vi "get property indeces.vi"(8 "error in":errorcluster, 10 "channels":refnum<class "TBM channel.lvclass">[](array[class]), 11 "data dictionary in":refnum<class "data dictionary.lvclass">) -> (0 "error out":errorcluster, 2 "File Property Indeces":i32[](array[numeric]), 3 "data dictionary out":refnum<class "data dictionary.lvclass">)   [LabVIEW 2015, in "TDMS datalogger runtime.lvclass"]
uses:
  TDMS datalogger runtime.lvclass
  <vilib>/NI/Tag Bus Module Framework/channel/TBM channel.lvclass
  <vilib>/NI/Tag Bus/dictionary/data dictionary.lvclass
  <vilib>/NI/Tag Bus/tag/tag descriptor.lvclass/tag descriptor.ctl
  <vilib>/NI/Tag Bus/tag/read tag name.vi
  <vilib>/NI/Tag Bus/tag/read data type.vi
  <vilib>/NI/Tag Bus/dictionary/locate tag.vi
  <vilib>/NI/Tag Bus/tag/tag descriptor.lvclass
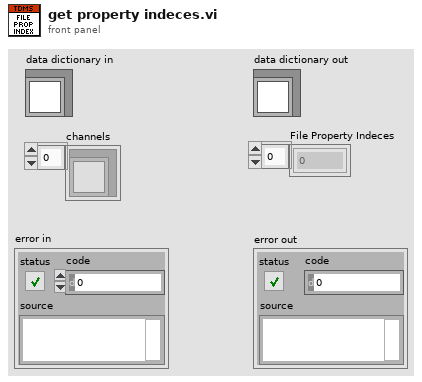
[diagram p1: front panel]
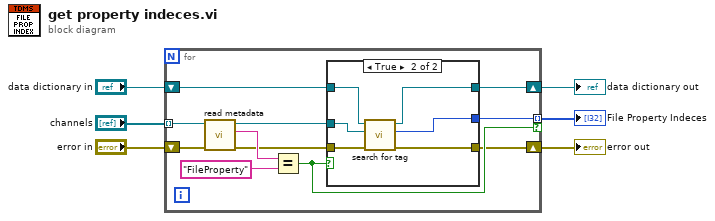
[diagram p0: block diagram]
diagram:
  n1 = for {
    tunnel: "channels" -> [w15] mode=indexing
    tunnel: [w10] -> w3 mode=indexing if=w13
    shift-right: [w9] -> w2
    shift-left: "data dictionary in" -> [w11]
    shift-right: [w7] -> w1
    shift-left: "error in" -> [w14]
    n2 = call <vilib>:"read metadata.vi"("error in"=w14, "system tag in"=w15) -> ("error out"=w8:errorcluster, "metadata"=w17:string, "system tag out"=w12:refnum<class "TBM channel.lvclass">)  [unwired: 7 in]
    n3 = Equal?(x=w17, y="FileProperty") -> (x = y?=w13:bool)
    n4 = case shown="True" w13 {
      tunnel: w12 -> [_ w25]
      tunnel: w11 -> [w19 w24]
      tunnel: [_ w23] -> w10
      tunnel: [w19 w22] -> w9
      tunnel: w8 -> [w18 w21]
      tunnel: [w18 w20] -> w7
      frame False {
      }
      frame True {
        n5 = call <vilib>:"search for tag.vi"("error in"=w21, "system tag"=w25, "data dictionary in"=w24) -> ("error out"=w20:errorcluster, "index"=w23:i32, "data dictionary out"=w22:refnum<class "data dictionary.lvclass">)  [unwired: 6 in]
      }
    }
  }
  "File Property Indeces" <- w3
  "data dictionary out" <- w2
  "error out" <- w1
